vi "PXI AO Write Delay.vi"(8 "error in (no error)":errorcluster) -> (0 "error out":errorcluster)   [LabVIEW 2015]
uses:
  PXI Globals.vi
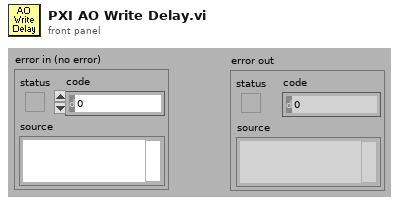
[diagram p1: front panel]
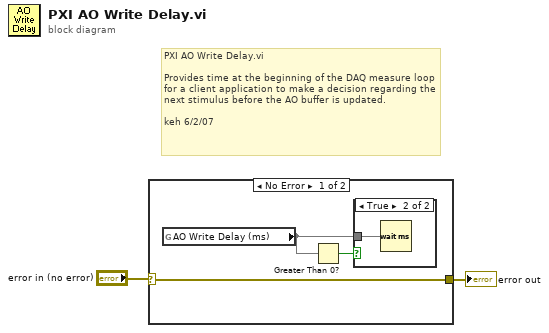
[diagram p0: block diagram]
diagram:
  # "PXI AO Write Delay.vi\n\nProvides time at the beginning of the DAQ measure loop for a client application to make a decision regarding the next stimulus before the AO buffer is updated.\n\nkeh 6/2/07"
  n1 = case shown="No Error" "error in (no error)" {
    selector: "error in (no error)" -> [w5 w7]
    tunnel: [w5 w7] -> w1
    frame No Error {
      n2 = global read "PXI Globals.vi" "AO Write Delay (ms)"() -> (w4)
      n3 = Greater Than 0?(x=w4) -> (x > 0?=w3:bool)
      n4 = case shown="True" w3 {
        tunnel: w4 -> [_ w6]
        frame False {
        }
        frame True {
          n5 = Wait (ms)(milliseconds to wait=w6) -> ()  [unwired: 1 out]
        }
      }
    }
    frame Error {
    }
  }
  "error out" <- w1
